vi "Frequency Sweep.vi"() -> ()   [LabVIEW 2020]
uses:
  <vilib>/Analysis/1siggen.llb/Ramp Pattern by Samples.vi
  <vilib>/DAQmx/write.llb/DAQmx Write (Analog Wfm 1Chan NSamp).vi
  <vilib>/DAQmx/create/channels.llb/DAQmx Create Channel (AO-Voltage-Basic).vi
  <vilib>/DAQmx/configure/timing.llb/DAQmx Timing (Sample Clock).vi
  <vilib>/DAQmx/miscellaneous.llb/DAQmx Fill In Error Info.vi
  <vilib>/measure/NI_MABase.lvlib
  <vilib>/Analysis/NI_AALBase.lvlib
panel:
  out "Current\nFrequency (Hz)":dbl
  in  "Number of\nSweep Samples":dbl
  in  "End Frequency (Hz)":dbl
  in  "Start Frequency (Hz)":dbl
  in  "Waveform Type":u16(ring) items=["Sine Wave", "Triangle Wave", "Square Wave", "Sawtooth Wave"]
  in  "Amplitude (Vp)":dbl=1.0 format="%0.2p"
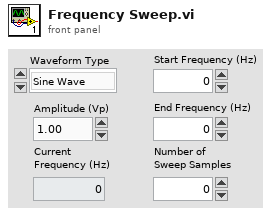
[diagram p1: front panel]
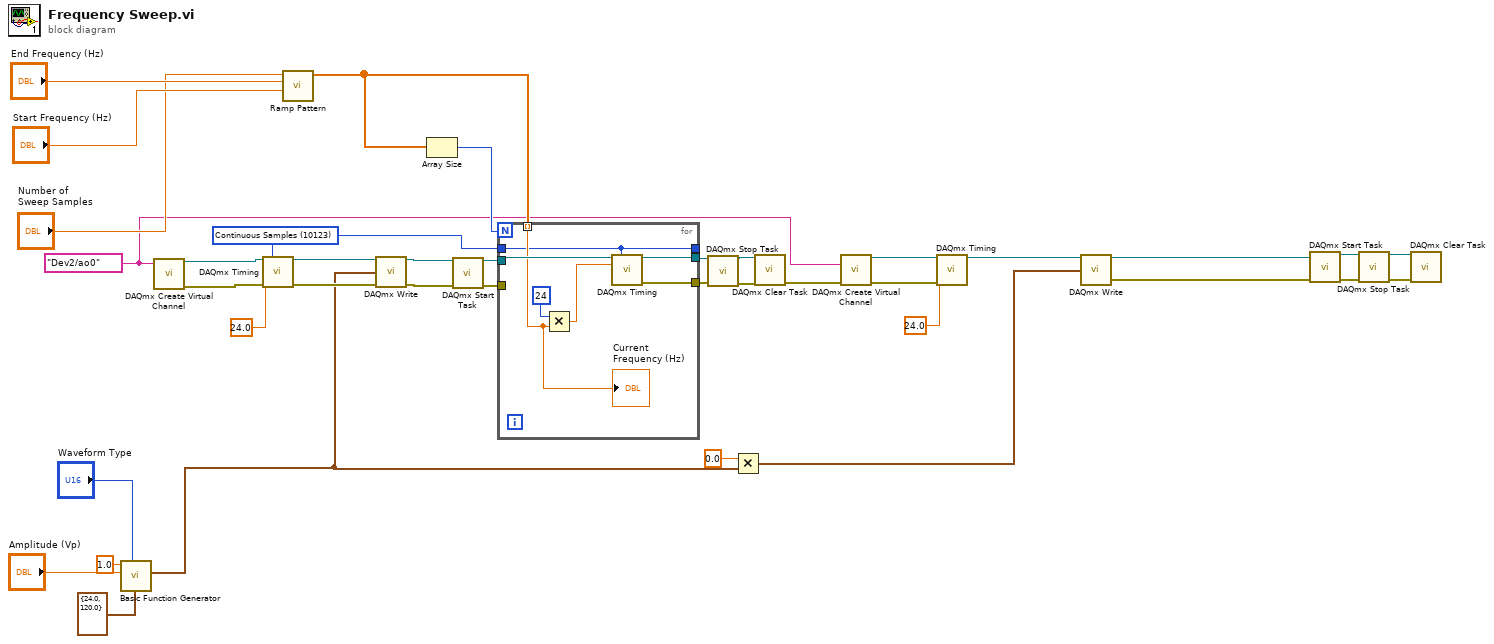
[diagram p0: block diagram]
diagram:
  w18 = 10123 items=["Finite Samples"=10178, "Continuous Samples"=10123, "Hardware Timed Single Point"=12522] ("sample mode")
  w1 = tag "Dev2/ao0" ("physical channels")
  n1 = call <vilib>:"Basic Function Generator.vi"("sampling info"=cluster{"Fs":dbl, "#s":dbl} {"Fs"=24.0, "#s"=120.0}, "signal type"="Waveform Type", "amplitude"="Amplitude (Vp)", "frequency"=1.0) -> ("signal out"=w27:waveform(dbl))  [unwired: 5 in, 2 out]
  n2 = call-poly <vilib>:"DAQmx Create Virtual Channel.vi"("physical channels"=w1) -> ("task out"=w38:refnum<k21>, "error out"=w37:errorcluster)  [unwired: 13 in]
  n3 = call-poly <vilib>:"DAQmx Timing.vi"("task/channels in"=w38, "sample mode"=w18, "rate"=24.0, "error in"=w37) -> ("task out"=w36:refnum<k21>, "error out"=w35:errorcluster)  [unwired: 10 in]
  n4 = call-poly <vilib>:"Ramp Pattern.vi"("start"="Start Frequency (Hz)", "end"="End Frequency (Hz)", "samples"="Number of\nSweep Samples") -> ("Ramp Pattern"=w20:dbl[])  [unwired: 7 in, 1 out]
  n5 = call-poly <vilib>:"DAQmx Write.vi"("task/channels in"=w36, "data"=w27, "error in"=w35) -> ("task out"=w33:refnum<k21>, "error out"=w32:errorcluster)  [unwired: 10 in, 1 out]
  n6 = Array Size(array=w20) -> (size(s)=w19:i32)
  n7 = call <vilib>:"DAQmx Start Task.vi"("task/channels in"=w33, "error in"=w32) -> ("task out"=w31:refnum<k21>, "error out"=w30:errorcluster)  [unwired: 12 in]
  n8 = for {
    N: w19 -> [_]
    tunnel: w31 -> [w44]
    tunnel: w30 -> [_]
    tunnel: [w45] -> w8
    tunnel: w20 -> [w41] mode=indexing
    tunnel: w18 -> [w40]
    tunnel: [w40] -> _
    tunnel: [w39] -> w9
    n9 = Multiply(x=24, y=w41) -> (x*y=w42:dbl)
    n10 = call-poly <vilib>:"DAQmx Timing.vi"("task/channels in"=w44, "sample mode"=w40, "rate"=w42) -> ("task out"=w45:refnum<k21>, "error out"=w39:errorcluster)  [unwired: 11 in]
    "Current\nFrequency (Hz)" <- w41
  }
  n11 = call <vilib>:"DAQmx Stop Task.vi"("task/channels in"=w8, "error in"=w9) -> ("task out"=w7:refnum<k21>, "error out"=w6:errorcluster)  [unwired: 12 in]
  n12 = Multiply(x=0.0, y=w27) -> (x*y=w10:waveform(dbl))
  n13 = call <vilib>:"DAQmx Clear Task.vi"("task in"=w7, "error in"=w6) -> ("error out"=w4:errorcluster)  [unwired: 13 in]
  n14 = call-poly <vilib>:"DAQmx Create Virtual Channel.vi"("physical channels"=w1, "error in"=w4) -> ("task out"=w13:refnum<k21>, "error out"=w3:errorcluster)  [unwired: 12 in]
  n15 = call-poly <vilib>:"DAQmx Timing.vi"("task/channels in"=w13, "rate"=24.0, "error in"=w3) -> ("task out"=w11:refnum<k21>)  [unwired: 11 in, 1 out]
  n16 = call-poly <vilib>:"DAQmx Write.vi"("task/channels in"=w11, "data"=w10) -> ("task out"=w5:refnum<k21>, "error out"=w2:errorcluster)  [unwired: 11 in, 1 out]
  n17 = call <vilib>:"DAQmx Start Task.vi"("task/channels in"=w5, "error in"=w2) -> ("task out"=w17:refnum<k21>, "error out"=w16:errorcluster)  [unwired: 12 in]
  n18 = call <vilib>:"DAQmx Stop Task.vi"("task/channels in"=w17, "error in"=w16) -> ("task out"=w15:refnum<k21>, "error out"=w14:errorcluster)  [unwired: 12 in]
  n19 = call <vilib>:"DAQmx Clear Task.vi"("task in"=w15, "error in"=w14) -> ()  [unwired: 13 in, 1 out]
